vi "TCP.IP Client for Ripple Detection_maybe.vi"() -> ()   [LabVIEW 2021]
doc: "Demonstrates how to open a connection to an TCP server, read the data being sent, and display the data on a chart. This VI is designed to stop if the TCP connection is terminated."
uses:
  <vilib>/Analysis/3filter.llb/Butterworth Filter (DBL).vi
  <vilib>/ptbypt/NI_PtbyPt.lvlib
  <vilib>/Analysis/NI_AALBase.lvlib
panel:
  in  "File Name":path=path "F:/Career/Work/From Now/Book2.csv"
  out "Filtered":dbl[](graph)
  out "Array Size 3":u32
  out "Delayed RMS2>RMS1 for 3 data":dynamicdata(graph)
  out "RMS2>RMS1 for 3 data":dynamicdata(graph)
  out "Array Size":u32
  out "RMS2>RMS1":dynamicdata(graph)
  out "RMS1":dynamicdata(graph)
  out "RMS2":dynamicdata(graph)
  out "Raw Data Collected":dynamicdata(graph)
  in  "Boolean":bool
  in  "Server Closed":string="The server VI closed the connection."
  out "Raw Data":dbl[](graph)
  in  "Stop":bool
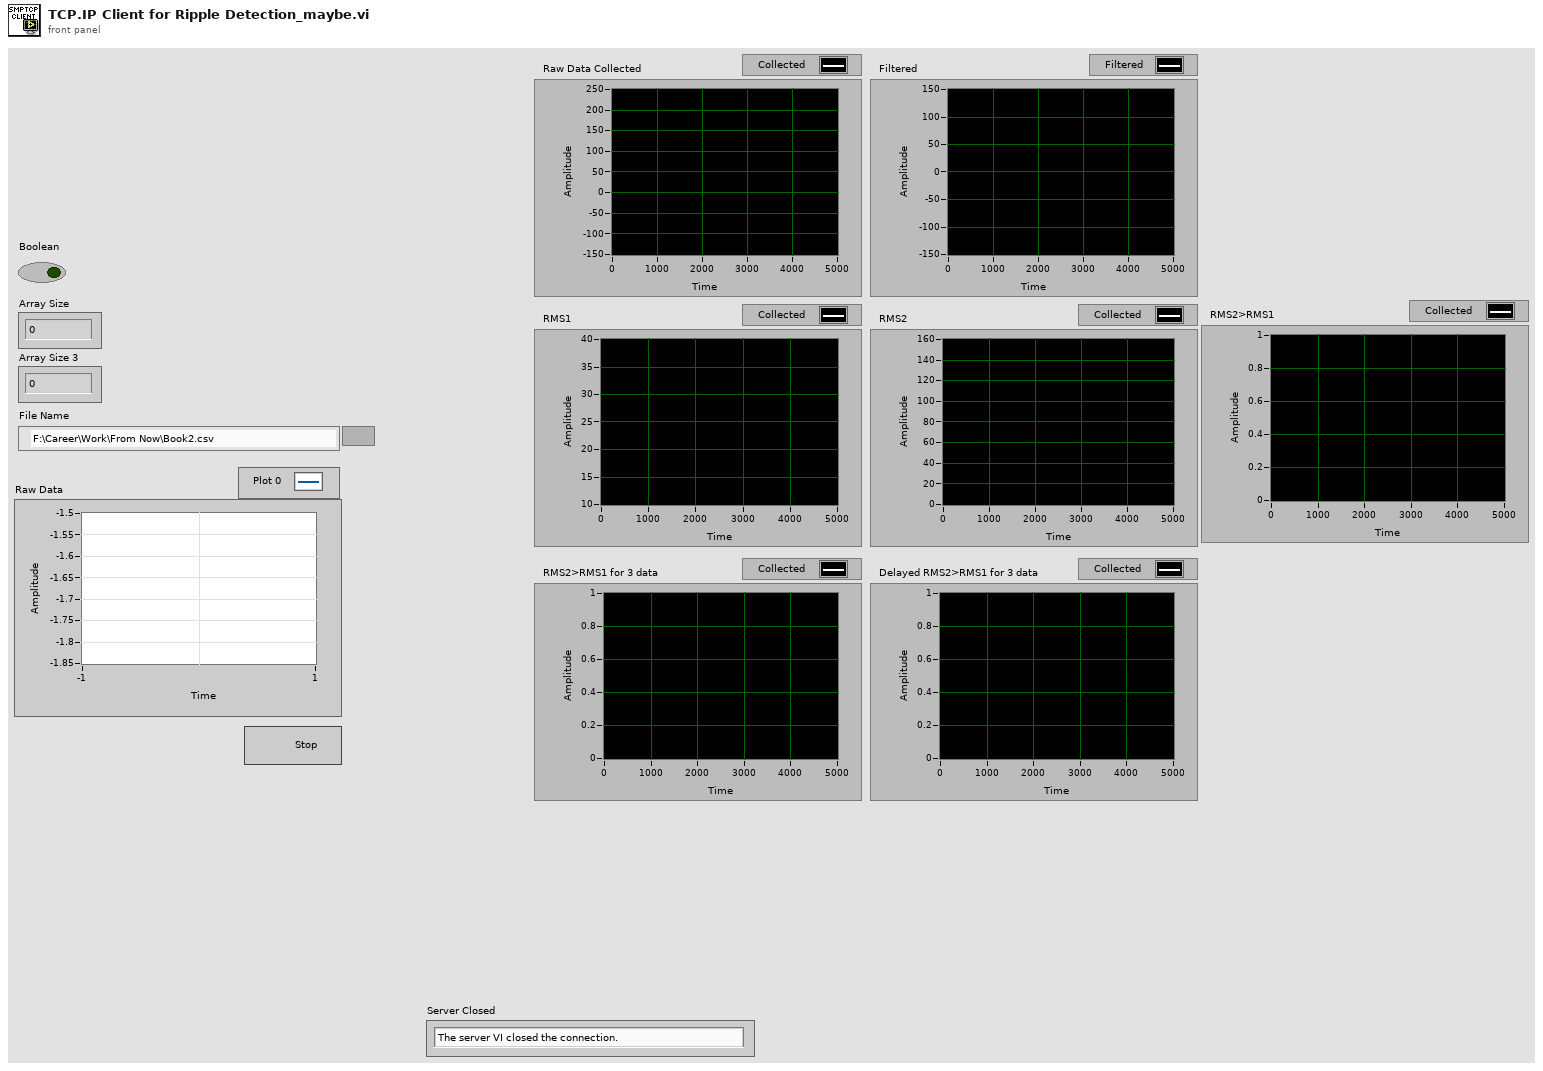
[diagram p1: front panel]
types:
  T1 = enum16{"open", "replace", "create", "open or create", "replace or create", "replace or create with confirmation"}
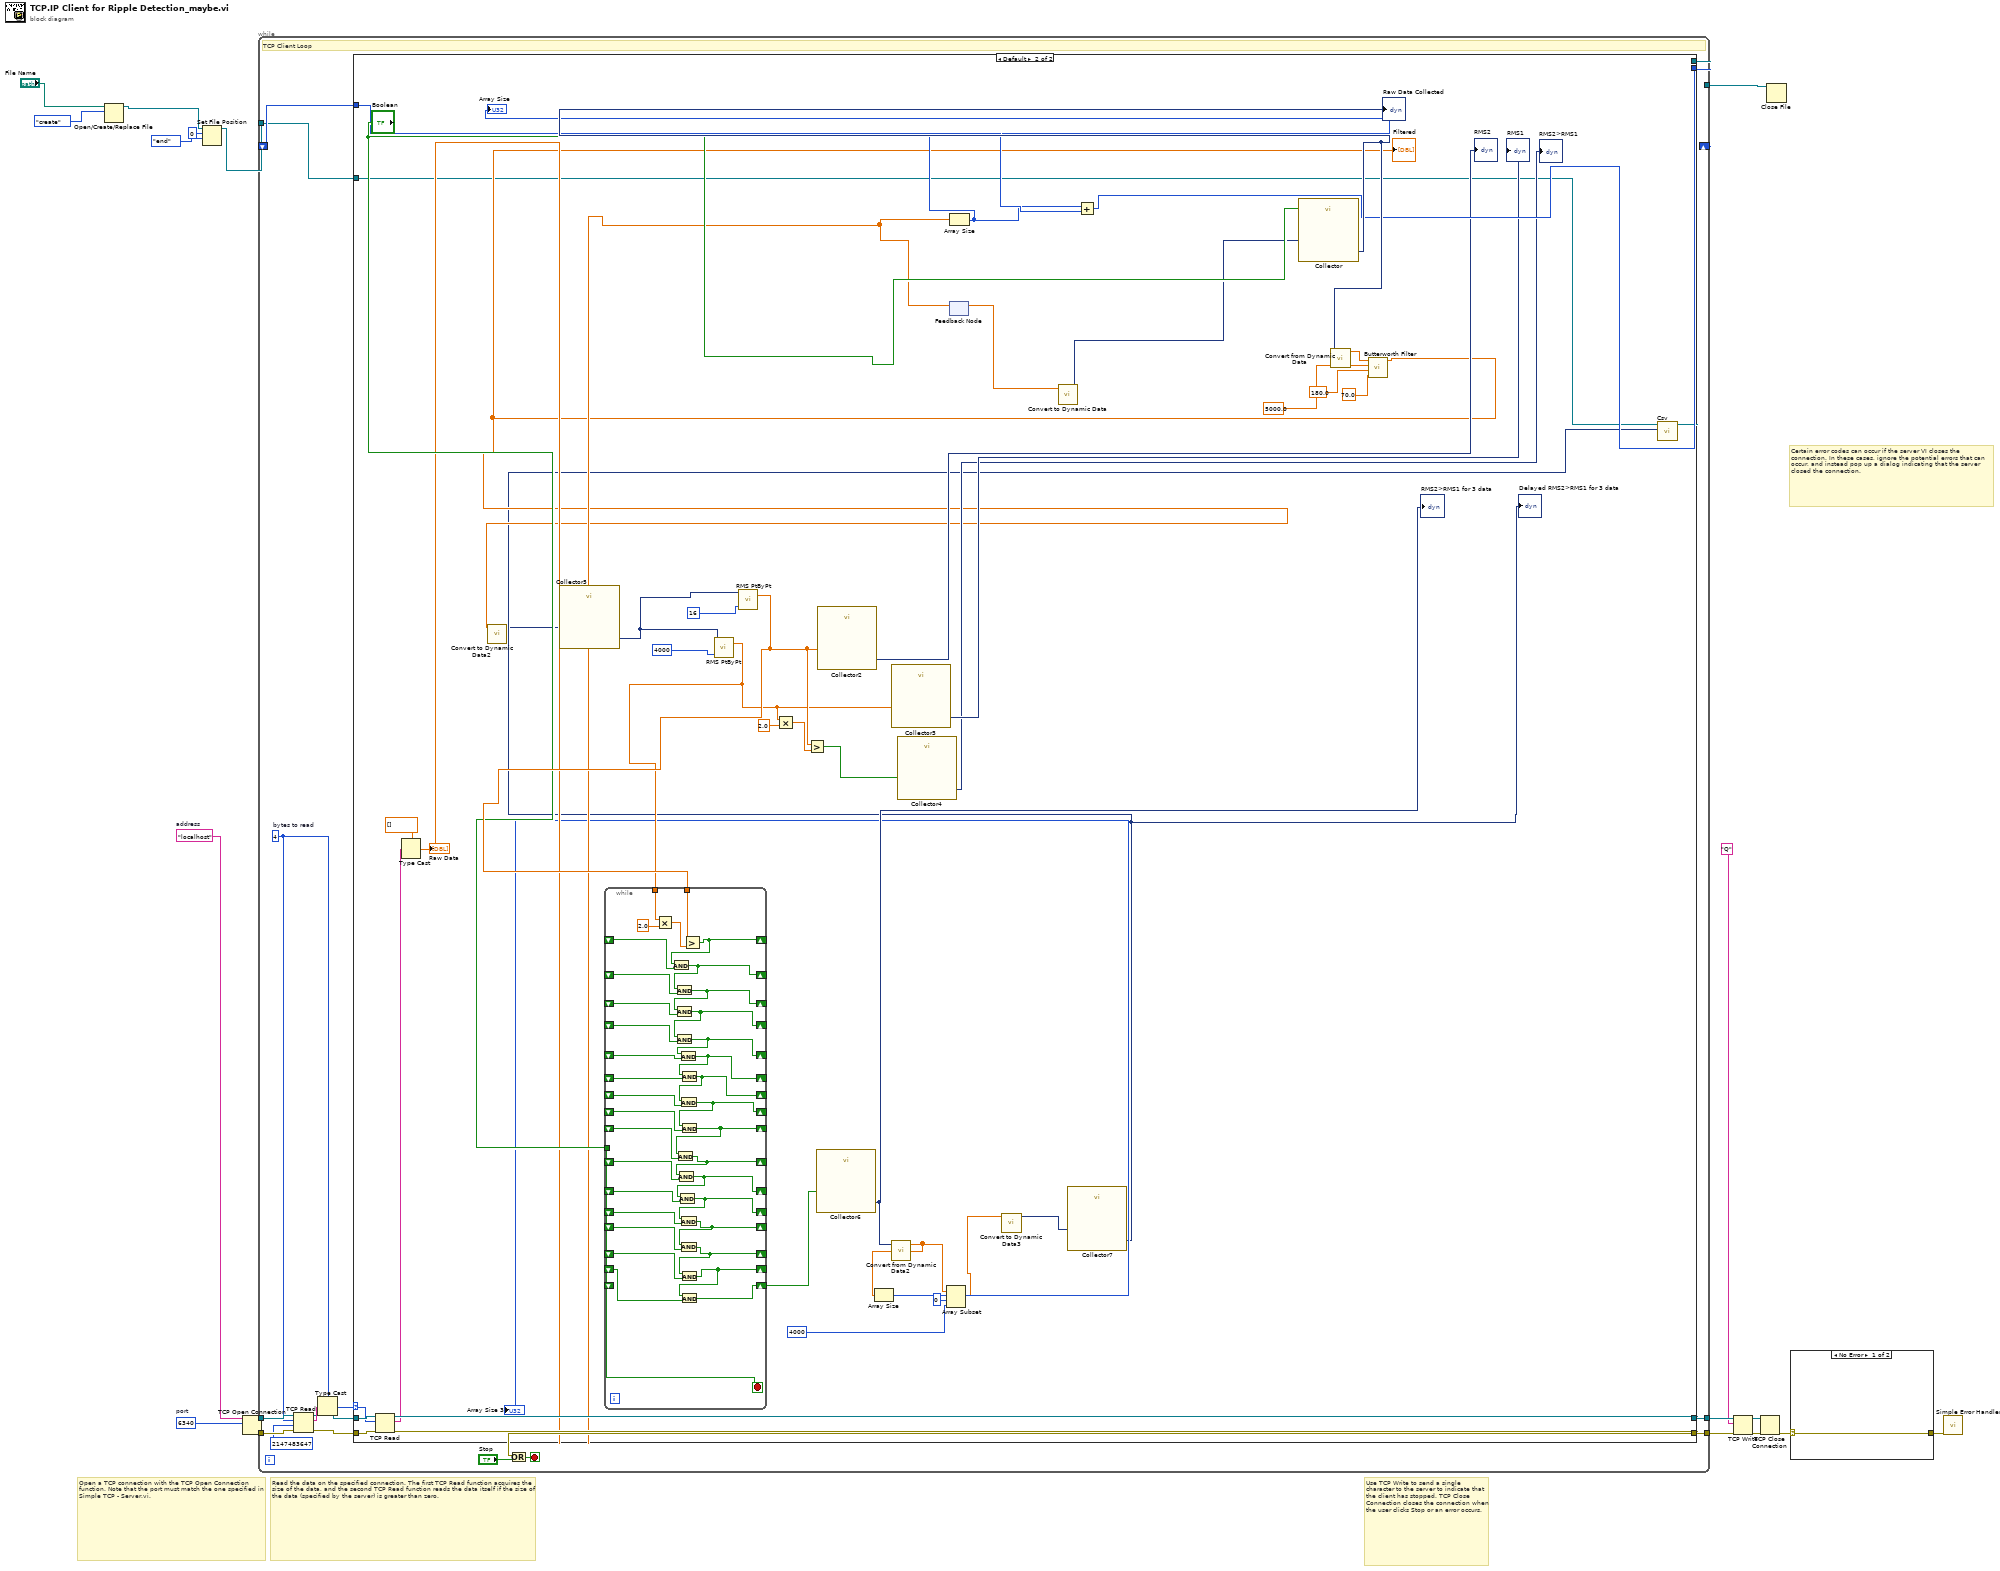
[diagram p0: block diagram]
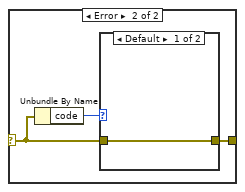
[diagram p2: hidden frame]
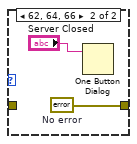
[diagram p3: hidden frame]
diagram:
  w8 = u16 6340  # port
  w9 = "localhost"  # address
  # "Certain error codes can occur if the server VI closes the connection. In these cases, ignore the potential errors that can occur, and instead pop up a dialog indicating that the server closed the connection."
  # "Use TCP Write to send a single character to the server to indicate that the client has stopped. TCP Close Connection closes the connection when the user clicks Stop or an error occurs."
  # "Read the data on the specified connection. The first TCP Read function acquires the size of the data, and the second TCP Read function reads the data itself if the size of the data (specified by the server) is greater than zero."
  # "Open a TCP connection with the TCP Open Connection function. Note that the port must match the one specified in Simple TCP - Server.vi."
  n1 = Open/Create/Replace File(file path (use dialog)="File Name", operation (0:open)=T1."create") -> (refnum out=w2:refnum<file>)  [unwired: 4 in, 2 out]
  n2 = Set File Position(offset (in bytes) (0)=i64 0, refnum=w2, from (0:start)=enum16{"start", "end", "current"}."end") -> (refnum out=w1:refnum<file>)  [unwired: 1 in, 1 out]
  n3 = TCP Open Connection(address=w9, remote port or service name=w8) -> (connection ID=w18:refnum<k5>, error out=w17:errorcluster)  [unwired: 3 in]
  n4 = while {
    tunnel: w17 -> [w30]
    tunnel: w18 -> [w31]
    tunnel: [w26] -> w15
    tunnel: [w25] -> w13
    shift-right: [w21] -> _
    shift-left: _ -> [w22]
    tunnel: [w20] -> w7
    tunnel: w1 -> [w19]
    stop <- w27 stop-if-true
    w29 = 4  # bytes to read
    # "TCP Client Loop"
    n5 = TCP Read(connection ID=w31, bytes to read=w29, error in (no error)=w30, 9:2147483647 ("timeout ms (25000)")) -> (connection ID out=w33:refnum<k5>, data out=w34:string, error out=w32:errorcluster)  [unwired: 1 in]
    n6 = Type Cast(type=w29, x=w34) -> (*(type *) &x=w24:i32)
    n7 = case shown="Default" w24 {
      selector: w24 -> [_ w75]
      tunnel: w33 -> [w38 w81]
      tunnel: w32 -> [w37 w80]
      tunnel: [w38 w78] -> w26
      tunnel: [w37 w77] -> w25
      tunnel: w22 -> [w36 w70]
      tunnel: [w36 w69] -> w21
      tunnel: w19 -> [w35 w59]
      tunnel: [w35 w58] -> w20
      frame ..0 {
        # "The server has not written any data"
      }
      frame Default {
        n8 = TCP Read(connection ID=w81, bytes to read=w75, error in (no error)=w80) -> (connection ID out=w78:refnum<k5>, data out=w76:string, error out=w77:errorcluster)  [unwired: 2 in]
        n9 = Type Cast(type=dbl[] [] ("chart"), x=w76) -> (*(type *) &x=w68:dbl[])
        "Raw Data" <- w68
        n10 = feedback #1() -> (w52:dbl[])  [unwired: 1 in]
        n11 = feedback-in #1(w68) -> ()
        n12 = Array Size(array=w68) -> (size(s)=w67:i32)
        "Array Size" <- w67
        n13 = call "Convert to Dynamic Data"("Array"=w52) -> ("Dynamic Data Type"=w53:dynamicdata)  [unwired: 3 in]
        n14 = Add(x=w67, y=w70) -> (x+y=w69:i32)
        n15 = call "Collector"("Enable"="Boolean", "Signals"=w53) -> ("Collected Signals"=w74:dynamicdata)  [unwired: 8 in, 1 out]
        "Raw Data Collected" <- w74
        n16 = call "Convert from Dynamic Data"("Dynamic Data Type"=w74) -> ("Array"=w54:dbl[])  [unwired: 3 in]
        n17 = call-poly <vilib>:"Butterworth Filter.vi"("low cutoff freq: fl"=70.0, "high cutoff freq: fh"=180.0, "sampling freq: fs"=5000.0, "X"=w54) -> ("Filtered X"=w61:dbl[])  [unwired: 4 in, 1 out]
        "Filtered" <- w61
        n18 = call "Convert to Dynamic Data2"("Array"=w61) -> ("Dynamic Data Type"=w46:dynamicdata)  [unwired: 3 in]
        n19 = call "Collector5"("Signals"=w46) -> ("Collected Signals"=w45:dynamicdata)  [unwired: 9 in, 1 out]
        n20 = call <vilib>:"RMS PtByPt.vi"("sample length"=4000, "x"=w45) -> ("rms value"=w72:dbl)  [unwired: 2 in, 1 out]
        n21 = call <vilib>:"RMS PtByPt.vi"("sample length"=16, "x"=w45) -> ("rms value"=w73:dbl)  [unwired: 2 in, 1 out]
        n22 = while {
          tunnel: w73 -> [w115]
          tunnel: w72 -> [w114]
          shift-right: [w109] -> _
          shift-left: _ -> [w110]
          shift-right: [w112] -> _
          shift-left: _ -> [w111]
          tunnel: "Boolean" -> [w113]
          shift-right: [w107] -> _
          shift-left: _ -> [w108]
          shift-right: [w105] -> _
          shift-left: _ -> [w106]
          shift-right: [w104] -> _
          shift-left: _ -> [w103]
          shift-right: [w95] -> _
          shift-left: _ -> [w88]
          shift-right: [w100] -> _
          shift-left: _ -> [w99]
          shift-right: [w102] -> _
          shift-left: _ -> [w101]
          shift-right: [w97] -> _
          shift-left: _ -> [w98]
          shift-right: [w96] -> _
          shift-left: _ -> [w89]
          shift-right: [w94] -> _
          shift-left: _ -> [w87]
          shift-right: [w93] -> _
          shift-left: _ -> [w86]
          shift-right: [w92] -> _
          shift-left: _ -> [w85]
          shift-right: [w91] -> _
          shift-left: _ -> [w84]
          shift-right: [w90] -> _
          shift-left: _ -> [w83]
          shift-right: [w82] -> w39
          shift-left: _ -> [_]
          stop <- w113 stop-if-true
          n23 = Multiply(x=w114, y=2.0) -> (x*y=w116:dbl)
          n24 = Greater?(x=w115, y=w116) -> (0:w112:bool)
          n25 = And(x=w112, y=w111) -> (x .and. y?=w109:bool)
          n26 = And(x=w109, y=w110) -> (x .and. y?=w107:bool)
          n27 = And(x=w107, y=w108) -> (x .and. y?=w105:bool)
          n28 = And(x=w105, y=w106) -> (x .and. y?=w104:bool)
          n29 = And(x=w104, y=w103) -> (x .and. y?=w102:bool)
          n30 = And(x=w102, y=w101) -> (x .and. y?=w100:bool)
          n31 = And(x=w100, y=w99) -> (x .and. y?=w97:bool)
          n32 = And(x=w97, y=w98) -> (x .and. y?=w96:bool)
          n33 = And(x=w96, y=w89) -> (x .and. y?=w95:bool)
          n34 = And(x=w95, y=w88) -> (x .and. y?=w94:bool)
          n35 = And(x=w94, y=w87) -> (x .and. y?=w93:bool)
          n36 = And(x=w93, y=w86) -> (x .and. y?=w92:bool)
          n37 = And(x=w92, y=w85) -> (x .and. y?=w91:bool)
          n38 = And(x=w91, y=w84) -> (x .and. y?=w90:bool)
          n39 = And(x=w90, y=w83) -> (x .and. y?=w82:bool)
        }
        n40 = Multiply(x=w72, y=2.0) -> (x*y=w48:dbl)
        n41 = Greater?(x=w73, y=w48) -> (0:w47:bool)
        n42 = call "Collector6"("Signals"=w39) -> ("Collected Signals"=w63:dynamicdata)  [unwired: 9 in, 1 out]
        "RMS2>RMS1 for 3 data" <- w63
        n43 = call "Collector2"("Signals"=w73) -> ("Collected Signals"=→"RMS2":dynamicdata)  [unwired: 9 in, 1 out]
        n44 = call "Collector3"("Signals"=w72) -> ("Collected Signals"=→"RMS1":dynamicdata)  [unwired: 9 in, 1 out]
        n45 = call "Convert from Dynamic Data2"("Dynamic Data Type"=w63) -> ("Array"=w41:dbl[])  [unwired: 3 in]
        n46 = Array Size(array=w41) -> (size(s)=→"Array Size 3":i32)
        n47 = call "Collector4"("Signals"=w47) -> ("Collected Signals"=→"RMS2>RMS1":dynamicdata)  [unwired: 9 in, 1 out]
        n48 = Array Subset(array=w41, index=0, length=4000 ("index")) -> (w40:dbl[])
        n49 = call "Convert to Dynamic Data3"("Array"=w40) -> ("Dynamic Data Type"=w44:dynamicdata)  [unwired: 3 in]
        n50 = call "Collector7"("Signals"=w44) -> ("Collected Signals"=w60:dynamicdata)  [unwired: 9 in, 1 out]
        "Delayed RMS2>RMS1 for 3 data" <- w60
        n51 = call "Csv.vi"("Delayed RMS2>RMS1 for 3 data"=w60, "Byte Stream File in"=w59) -> ("Byte Stream File out"=w58:refnum<file>)  [unwired: 9 in]
      }
    }
    n52 = Or(x=w25, y="Stop") -> (x .or. y?=w27:bool)
  }
  n53 = TCP Write(connection ID=w15, data in="Q", error in (no error)=w13) -> (connection ID out=w16:refnum<k5>, error out=w14:errorcluster)  [unwired: 2 out]
  n54 = TCP Close Connection(connection ID=w16, error in (no error)=w14) -> (error out=w11:errorcluster)  [unwired: 1 in, 1 out]
  n55 = Close File(refnum=w7) -> ()  [unwired: 1 in, 2 out]
  n56 = case shown="No Error" w11 {
    selector: w11 -> [w118 w120]
    tunnel: [w118 w119] -> w10
    frame No Error {
    }
    frame Error {
      n57 = Unbundle By Name(w120) -> ("code"=w121:i32)
      n58 = case shown="Default" w121 {
        tunnel: w120 -> [w122 _]
        tunnel: [w122 w124] -> w119
        frame Default {
        }
        frame 62, 64, 66 {
          w124 = errorcluster {"status"=FALSE, "code"=0, "source"=""}  # No error
          n59 = One Button Dialog(message="Server Closed") -> ()  [unwired: 1 in, 1 out]
        }
      }
    }
  }
  n60 = call <vilib>:"Simple Error Handler.vi"("error in (no error)"=w10) -> ()  [unwired: 4 in, 5 out]
